vi "Write to File.vi"(8 "error in":errorcluster, 11 "File Obs in":refnum<class "File Observer.lvclass">) -> (0 "error out":errorcluster, 3 "File Obs out":refnum<class "File Observer.lvclass">)   [LabVIEW 2015, in "File Observer.lvclass"]
doc: "Write data to the file indicated by the File Observer.File Reference property if there there is fresh data (i.e. the dequeue does not time out) and if the Write property == TRUE. If data is to be written, first check to make sure that the maximum file size has not been exceeded. If it has, close the current file reference and open a new one. Finally, write the data to the specified file."
uses:
  File Observer.lvclass
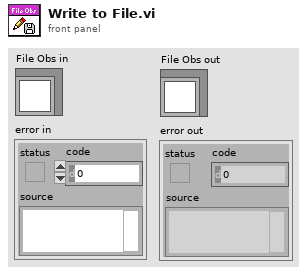
[diagram p1: front panel]
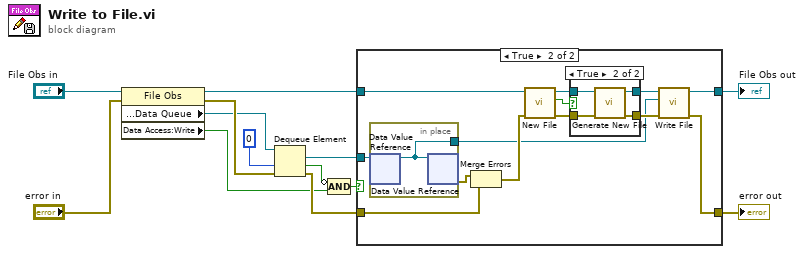
[diagram p0: block diagram]
diagram:
  n1 = property class="File Obs"(reference="File Obs in", error in="error in") -> (reference out=w1:refnum<class "File Observer.lvclass">, error out=w8:errorcluster, "Data Access:Data Queue"=w7:refnum<queue>, "Data Access:Write"=w2:bool)
  n2 = Dequeue Element(queue=w7, timeout in ms (-1)=0, error in (no error)=w8) -> (element=w6:refnum<data-value>, timed out?=w4:bool, error out=w5:errorcluster)  [unwired: 1 out]
  n3 = Compound Arithmetic op=AND(invert w4, w2) -> (w3:bool)
  n4 = case shown="True" w3 {
    tunnel: w6 -> [_ w18]
    tunnel: [w15 w22] -> w12
    tunnel: w5 -> [w15 w28]
    tunnel: w1 -> [w14 w20]
    tunnel: [w14 w24] -> w10
    frame False {
    }
    frame True {
      n5 = in-place {
        in-place-border: [w29] -> w16
        n6 = in-place-dvr #1(w18) -> (w29:refnum<class "Data.lvclass">)  [unwired: 1 out]
        n7 = in-place-dvr #1(w29) -> (w17:errorcluster)  [unwired: 1 out]
      }
      n8 = Merge Errors(w17, w28) -> (w27:errorcluster)
      n9 = call-dynamic "New File.vi"("error in"=w27, "File Observer in"=w20) -> ("error out"=w26:errorcluster, "Exceeded"=w21:bool, "File Observer out"=w19:refnum<class "File Observer.lvclass">)  [unwired: 7 in]
      n10 = case shown="True" w21 {
        tunnel: w19 -> [w31 w35]
        tunnel: [w31 w34] -> w25
        tunnel: w26 -> [w30 w33]
        tunnel: [w30 w32] -> w23
        frame False {
        }
        frame True {
          n11 = call-dynamic "Generate New File.vi"("error in"=w33, "File Obs in"=w35) -> ("error out"=w32:errorcluster, "File Obs out"=w34:refnum<class "File Observer.lvclass">)  [unwired: 7 in, 1 out]
        }
      }
      n12 = call-dynamic "Write File.vi"("error in"=w23, "Data In"=w16, "File Obs in"=w25) -> ("error out"=w22:errorcluster, "File Obs out"=w24:refnum<class "File Observer.lvclass">)  [unwired: 7 in]
    }
  }
  "error out" <- w12
  "File Obs out" <- w10
